vi "subVI Freq_Meas.vi"(1 "Filter Length":u8=8, 2 "Sampling Frequency":dbl format="%#_13g", 3 "Time Window":dbl format="%#_13g", 4 "Scaled Waveform":dbl[](array[numeric])) -> (0 "Signals":dbl[][](graph))   [LabVIEW 2022 SP3]
panel:
  out "Estimated Frequency":dbl
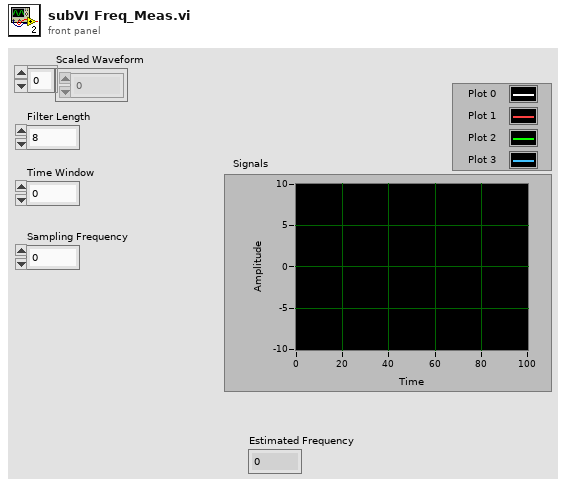
[diagram p1: front panel]
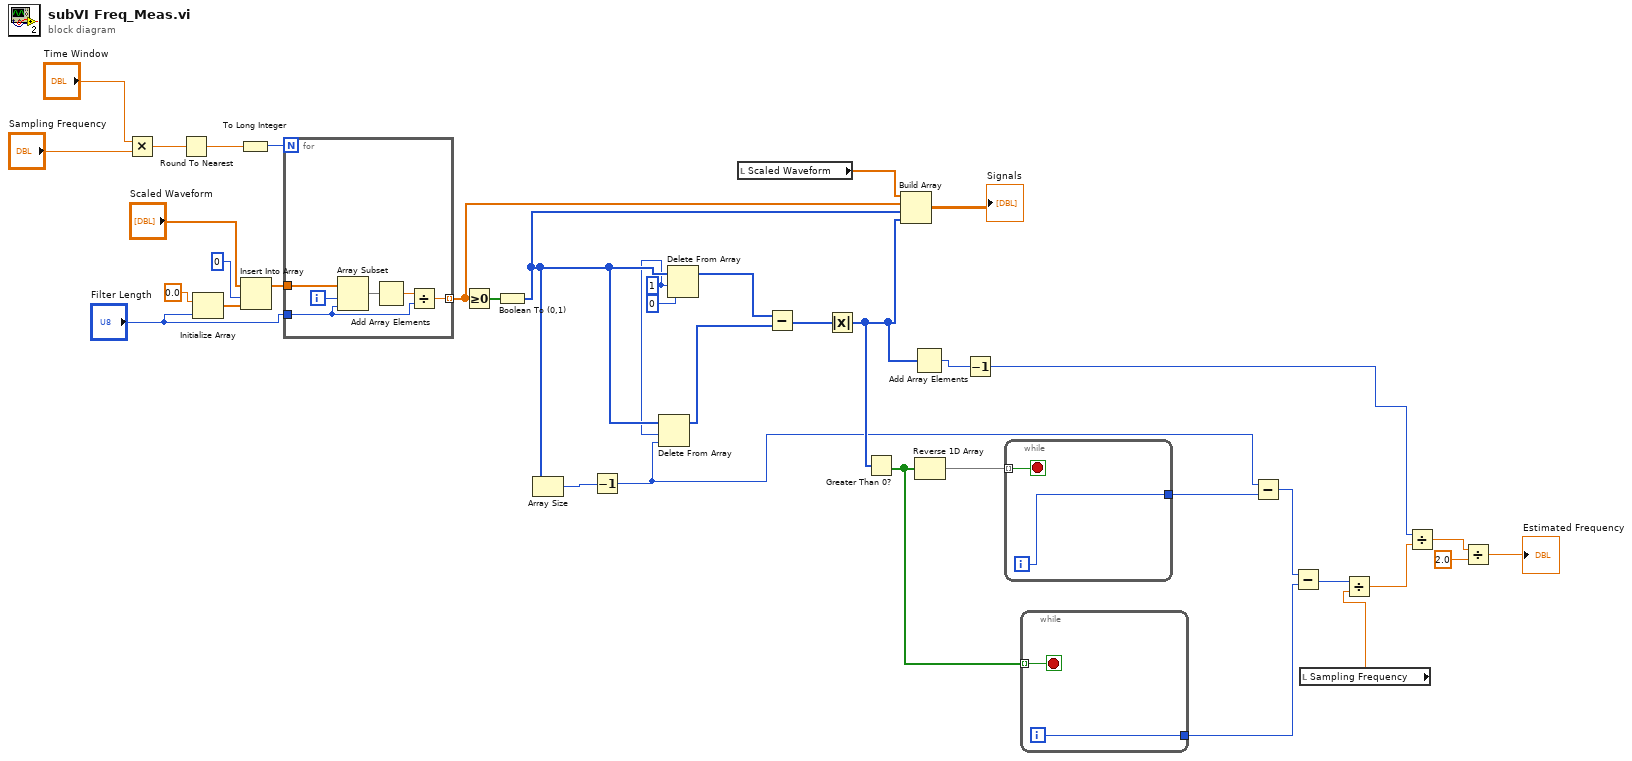
[diagram p0: block diagram]
diagram:
  w22 = 1 ("length")
  n1 = Multiply(x="Time Window", y="Sampling Frequency") -> (x*y=w36:dbl)
  n2 = Round To Nearest(number=w36) -> (nearest integer value=w35:dbl)
  n3 = Initialize Array(0.0 ("element"), "Filter Length") -> (w32:dbl[])
  n4 = To Long Integer(number=w35) -> (32bit integer=w34:i32)
  n5 = Insert Into Array(array="Scaled Waveform", index=0, new element=w32) -> (w30:dbl[])
  n6 = for {
    N: w34 -> [_]
    tunnel: w30 -> [w43]
    tunnel: "Filter Length" -> [w39]
    tunnel: [w38] -> w26 mode=indexing
    i -> [w42]
    n7 = Array Subset(array=w43, index=w42, length=w39) -> (w41:dbl[])
    n8 = Add Array Elements(numeric array=w41) -> (sum=w40:dbl)
    n9 = Divide(x=w40, y=w39) -> (x/y=w38:dbl)
  }
  n10 = Greater Or Equal To 0?(x=w26) -> (x >= 0?=w28:bool[])
  n11 = Boolean To (0,1)(Boolean=w28) -> (0, 1=w23:i16[])
  n12 = Array Size(array=w23) -> (size(s)=w24:i32)
  n13 = Decrement(x=w24) -> (x-1=w13:i32)
  n14 = Delete From Array(array=w23, length=w22, index=w13) -> (array with subset deleted=w20:i16[])  [unwired: 1 out]
  n15 = Delete From Array(array=w23, length=w22, index=0) -> (array with subset deleted=w21:i16[])  [unwired: 1 out]
  n16 = local read "Scaled Waveform"() -> (w1:dbl[])
  n17 = Subtract(x=w21, y=w20) -> (x-y=w19:i16[])
  n18 = Absolute Value(x=w19) -> (abs(x)=w16:i16[])
  n19 = Greater Than 0?(x=w16) -> (x > 0?=w14:bool[])
  n20 = Build Array(w1, w26, w23, w16) -> (→"Signals":dbl[][])
  n21 = Add Array Elements(numeric array=w16) -> (sum=w17:i16)
  n22 = Reverse 1D Array(array=w14) -> (reversed array=w15:bool[])
  n23 = Decrement(x=w17) -> (x-1=w2:i16)
  n24 = while {
    tunnel: w15 -> [w45] mode=indexing
    tunnel: [w44] -> w12
    i -> [w44]
    stop <- w45 stop-if-true
  }
  n25 = while {
    tunnel: w14 -> [w47] mode=indexing
    tunnel: [w46] -> w10
    i -> [w46]
    stop <- w47 stop-if-true
  }
  n26 = Subtract(x=w13, y=w12) -> (x-y=w11:i32)
  n27 = Subtract(x=w11, y=w10) -> (x-y=w9:i32)
  n28 = local read "Sampling Frequency"() -> (w3:dbl)
  n29 = Divide(x=w9, y=w3) -> (x/y=w7:dbl)
  n30 = Divide(x=w2, y=w7) -> (x/y=w6:dbl)
  n31 = Divide(x=w6, y=2.0) -> (x/y=→"Estimated Frequency":dbl)
